vi "(BASVR) Choose Range.vi"(6 "error in (no error)":errorcluster, 8 "Group Name":string, 10 "Chosen Channel":i32, 11 "tdms ref":refnum<k34>) -> (2 "Chosen Range":u8, 4 "error out":errorcluster)   [LabVIEW 2023]
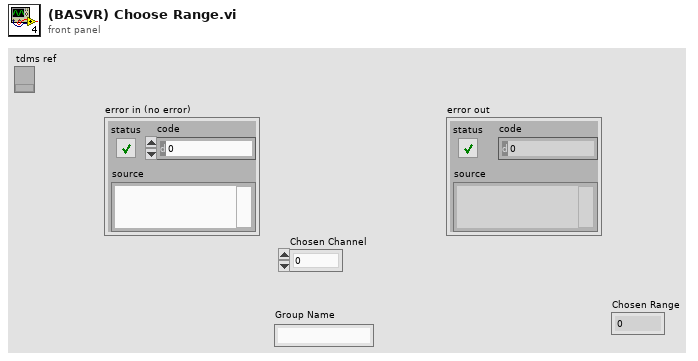
[diagram p1: front panel]
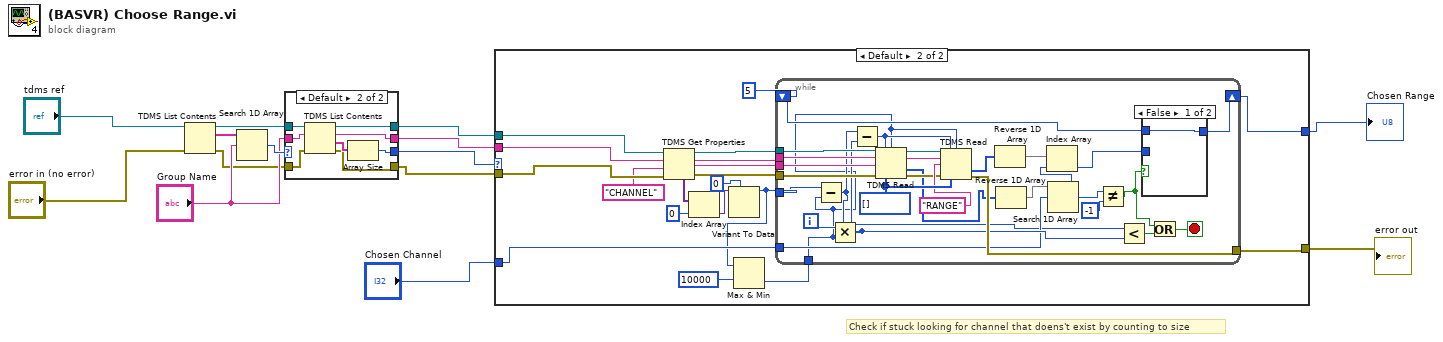
[diagram p0: block diagram]
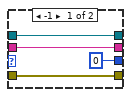
[diagram p2: hidden frame]
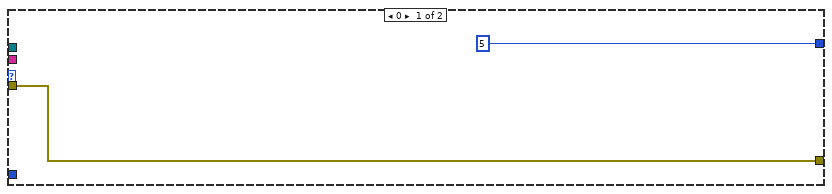
[diagram p3: hidden frame]
diagram:
  # "Check if stuck looking for channel that doens't exist by counting to size"
  n1 = TDMS List Contents(4:"error in (no error)", 7:"tdms ref") -> (0:w5:errorcluster, 2:w10:string[], 3:w9:refnum<k34>)  [unwired: 1 in, 1 out]
  n2 = Search 1D Array(1D array=w10, element="Group Name") -> (index of element=w8:i32)  [unwired: 1 in]
  n3 = case shown="Default" w8 {
    tunnel: [w17 w26] -> w12
    tunnel: [w16 w25] -> w11
    tunnel: [0 w23] -> w7
    tunnel: w9 -> [w17 w22]
    tunnel: "Group Name" -> [w16 w21]
    tunnel: w5 -> [w15 w20]
    tunnel: [w15 w19] -> w4
    frame -1 {
    }
    frame Default {
      n4 = TDMS List Contents(4:w20, 6:w21, 7:w22) -> (0:w19:errorcluster, 1:w24:string[], 2:w25:string, 3:w26:refnum<k34>)
      n5 = Array Size(array=w24) -> (size(s)=w23:i32)
    }
  }
  n6 = case shown="Default" w7 {
    tunnel: "Chosen Channel" -> [_ w47]
    tunnel: [5 w46] -> w13
    tunnel: w11 -> [_ w43]
    tunnel: w12 -> [_ w44]
    tunnel: w4 -> [w27 w42]
    tunnel: [w27 w36] -> w2
    frame 0 {
    }
    frame Default {
      n7 = TDMS Get Properties(8:w42, 9:"CHANNEL" ("Channel Track"), 10:w43, 11:w44) -> (0:w37:errorcluster, 1:w38:string, 2:w40:string, 3:w41:refnum<k34>, 4:w35:variant[])  [unwired: 2 in, 1 out]
      n8 = Index Array(array=w35, index=0) -> (element=w33:variant)
      n9 = Variant To Data(type=0, Variant=w33) -> (data=w31:i32)  [unwired: 1 in, 1 out]
      n10 = Max & Min(x=w31, y=10000) -> (min(x,y)=w29:i32)  [unwired: 1 out]
      n11 = while {
        tunnel: w47 -> [w54]
        shift-right: [w63] -> w46
        shift-left: 5 -> [w76]
        tunnel: w41 -> [w73]
        tunnel: w40 -> [w72]
        tunnel: w38 -> [w71]
        tunnel: w37 -> [w70]
        tunnel: [w62] -> w36
        tunnel: w31 -> [w48]
        tunnel: w29 -> [w49]
        i -> [w61]
        stop <- w75 stop-if-true
        w68 = i32[] []
        n12 = Subtract(x=w48, y=w49) -> (x-y=w50:i32)
        n13 = Multiply(x=w61, y=w49) -> (x*y=w60:i32)
        n14 = Subtract(x=w50, y=w60) -> (x-y=w69:i32)
        n15 = TDMS Read(0:w73, 1:w69, 2:w49, 5:w72, 7:w71, 11:w70, 12:w68) -> (4:w65:refnum<k34>, 6:w66:string, 10:w59:i32[], 15:w64:errorcluster)  [unwired: 1 in, 2 out]
        n16 = TDMS Read(0:w65, 1:w69, 2:w49, 5:w66, 7:"RANGE" ("Channel Track"), 11:w64, 12:w68) -> (10:w58:i32[], 15:w62:errorcluster)  [unwired: 1 in, 4 out]
        n17 = Reverse 1D Array(array=w58) -> (reversed array=w53:i32[])
        n18 = Reverse 1D Array(array=w59) -> (reversed array=w57:i32[])
        n19 = Search 1D Array(1D array=w57, element=w54) -> (index of element=w52:i32)  [unwired: 1 in]
        n20 = Index Array(array=w53, index=w52) -> (element=w51:i32)
        n21 = Not Equal?(x=w52, y=-1) -> (x != y?=w56:bool)
        n22 = Less?(x=w50, y=w60) -> (x < y?=w74:bool)
        n23 = case shown="False" w56 {
          tunnel: w51 -> [_ w78]
          tunnel: [w77 w78] -> w63
          tunnel: w76 -> [w77 _]
          frame False {
          }
          frame True {
          }
        }
        n24 = Or(x=w56, y=w74) -> (x .or. y?=w75:bool)
      }
    }
  }
  "Chosen Range" <- w13
  "error out" <- w2
